vi "PathfinderUtil_Continuous_Heading_Difference.vi"(10 "Heading Diff":dbl) -> (2 "Heading Diff":dbl)   [LabVIEW 2019, in "Trajectory_Library.lvlib"]
doc: "Normalize a heading difference so that it falls withing (+/- PI)."
uses:
  Trajectory_Library.lvlib
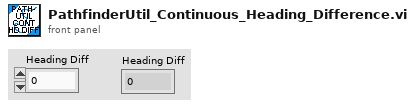
[diagram p1: front panel]
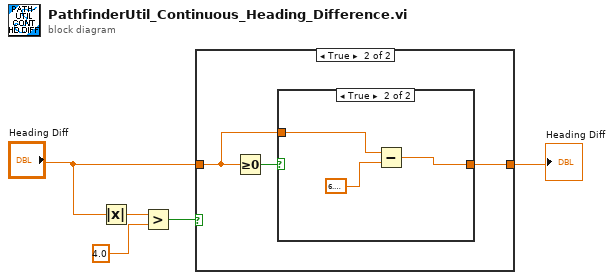
[diagram p0: block diagram]
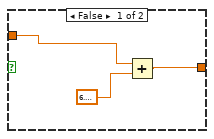
[diagram p3: hidden frame]
diagram:
  n1 = Absolute Value(x="Heading Diff") -> (abs(x)=w5:dbl)
  n2 = Greater?(x=w5, y=4.0) -> (0:w3:bool)
  n3 = case shown="True" w3 {
    tunnel: "Heading Diff" -> [w6 w8]
    tunnel: [w6 w7] -> w1
    frame False {
    }
    frame True {
      n4 = Greater Or Equal To 0?(x=w8) -> (x >= 0?=w9:bool)
      n5 = case shown="True" w9 {
        tunnel: w8 -> [w11 w14]
        tunnel: [w10 w13] -> w7
        frame False {
          n6 = Add(x=w11, y=6.283185307179586) -> (x+y=w10:dbl)
        }
        frame True {
          n7 = Subtract(x=w14, y=6.283185307179586) -> (x-y=w13:dbl)
        }
      }
    }
  }
  "Heading Diff" <- w1
